vi "Update Timer.vi"(8 "error in (no error)":errorcluster, 10 "Timer (s)":dbl, 11 "Kitchen Actor in":refnum<class "Kitchen Actor.lvclass">) -> (0 "error out":errorcluster, 3 "Kitchen Actor out":refnum<class "Kitchen Actor.lvclass">)   [LabVIEW 2024, in "Kitchen Actor.lvlib" / "Kitchen Actor.lvclass"]
uses:
  Kitchen Actor.lvclass
  Kitchen Actor.lvclass/Kitchen Actor.ctl
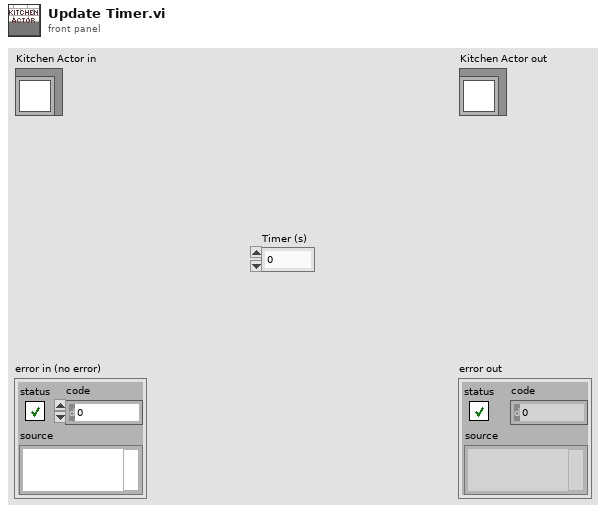
[diagram p1: front panel]
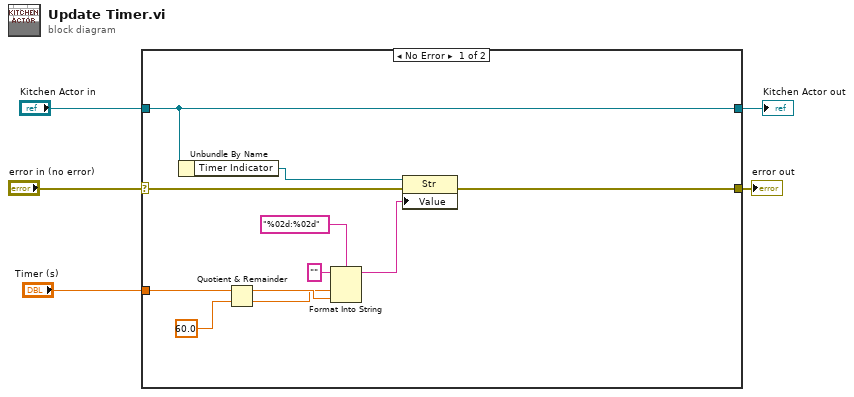
[diagram p0: block diagram]
diagram:
  n1 = case shown="No Error" "error in (no error)" {
    selector: "error in (no error)" -> [w16 w18]
    tunnel: [w14 w18] -> w4
    tunnel: [w15 w17] -> w2
    tunnel: "Kitchen Actor in" -> [w15 w17]
    tunnel: "Timer (s)" -> [w10 _]
    frame No Error {
      n2 = Unbundle By Name(w15) -> ("Timer Indicator"=w13:refnum<vi>)
      n3 = Quotient & Remainder(x=w10, y=60.0) -> (x-y*floor(x/y)=w8:dbl, floor(x/y)=w7:dbl)
      n4 = Format Into String(format string="%02d:%02d", initial string="", w7, w8) -> (resulting string=w12:string)  [unwired: 1 in, 1 out]
      n5 = property class="Str"(reference=w13, error in=w16, "Value"=w12) -> (error out=w14:errorcluster)  [unwired: 1 out]
    }
    frame Error {
    }
  }
  "error out" <- w4
  "Kitchen Actor out" <- w2
